vi "Test type to no.vi"(10 "String":string) -> (2 "number":dbl)   [LabVIEW 2011]
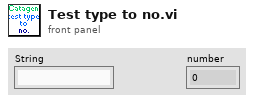
[diagram p1: front panel]
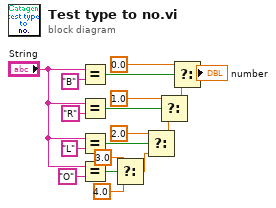
[diagram p0: block diagram]
diagram:
  n1 = Equal?(x="String", y="B") -> (x = y?=w11:bool)
  n2 = Equal?(x="String", y="R") -> (x = y?=w14:bool)
  n3 = Equal?(x="String", y="L") -> (x = y?=w6:bool)
  n4 = Equal?(x="String", y="O") -> (x = y?=w2:bool)
  n5 = Select(t=3.0, s=w2, f=4.0 ("t")) -> (s? t:f=w4:dbl)
  n6 = Select(t=2.0, s=w6, f=w4) -> (s? t:f=w18:dbl)
  n7 = Select(t=1.0, s=w14, f=w18) -> (s? t:f=w16:dbl)
  n8 = Select(t=0.0, s=w11, f=w16) -> (s? t:f=→"number":dbl)
